vi "Subvi for fastbox.vi"(0 "Cluster in":T1 {"Y axis\nrotation" scale=-32700.0..32700.0; "X axis\nrotation" scale=-32700.0..32700.0; "Z axis" scale=-32700.0..32700.0; "Y axis" scale=-32700.0..32700.0; "X axis" scale=-32700.0..32700.0}, 1 "FPGA VI Reference In":refnum<k20>) -> ()   [LabVIEW 2009]
uses:
  UPD Xbox.ctl
  <vilib>/rvi/interface/nirviReadWriteControl/nirviReadWriteControl.xnode
  FPGA Bitfiles/Athena Brain.lvproj_FPGA Target 2_Combined Steering ~2D.lvbitx
  <vilib>/Utility/error.llb/Error Cluster From Error Code.vi
  <vilib>/rvi/errors/niLvFpgaAdjustHostInterfaceError.vi
  <vilib>/rvi/interface/common/niFpgaNodeNameForErrorReporting.ctl
  <vilib>/rvi/errors/niLvFpgaWhatHappensToTopLevelVI.ctl
  NiRioSrv.dll
panel:
  out "Drive Encoder ft/sec":fxp<+/-,14,4> format="%.12g"
  out "Drive Encoder":i32
  out "Drive Encoder tick/count":i32
  in  "Steering Position Offset":i32
  in  "Steering Proportional Control Feedback Gain":fxp<+/-,20,5> format="%.17g"
  in  "Scale the Steering":dbl
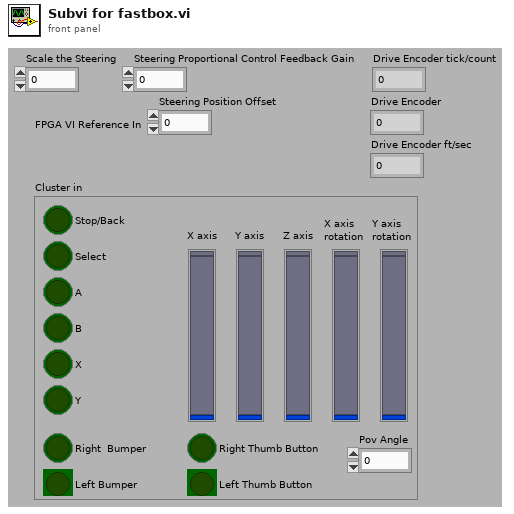
[diagram p1: front panel]
types:
  T1 = typedef "UPD Xbox.ctl" = cluster{"B":bool, "A":bool, "Y":bool, "X":bool, "X axis":i32, "Y axis":i32, "Z axis":i32, "X axis\nrotation":i32, "Y axis\nrotation":i32, "Left Bumper":bool, "Right  Bumper":bool, "Left Thumb Button":bool, "Right Thumb Button":bool, "Stop/Back":bool, "Select":bool, "Pov Angle":i32}
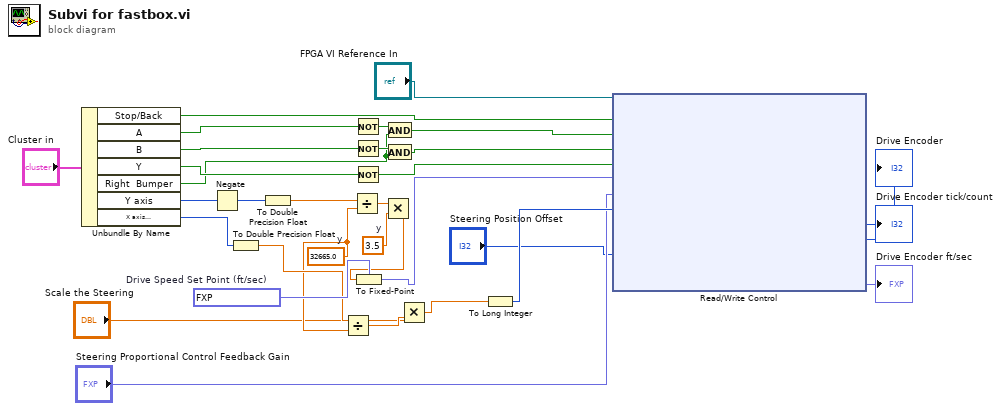
[diagram p0: block diagram]
diagram:
  w11 = 3.5  # y
  w12 = 32665.0  # y
  w29 = fxp<+/-,14,4> 0.0  # Drive Speed Set Point (ft/sec)
  n1 = Unbundle By Name("Cluster in") -> ("Stop/Back"=w31:bool, "A"=w20:bool, "B"=w21:bool, "Y"=w27:bool, "Right  Bumper"=w22:bool, "Y axis"=w30:i32, "X axis\nrotation"=w14:i32)
  n2 = Negate(x=w30) -> (-x=w1:i32)
  n3 = To Double Precision Float(number=w14) -> (double precision float=w13:dbl)
  n4 = To Double Precision Float(number=w1) -> (double precision float=w15:dbl)
  n5 = Divide(x=w13, y=w12) -> (x/y=w10:dbl)
  n6 = Divide(x=w15, y=w12) -> (x/y=w32:dbl)
  n7 = Not(x=w20) -> (.not. x?=w23:bool)
  n8 = Not(x=w21) -> (.not. x?=w24:bool)
  n9 = Not(x=w27) -> (.not. x?=w28:bool)
  n10 = Multiply(x=w32, y=w11) -> (x*y=w17:dbl)
  n11 = To Fixed-Point(fixed-point type=w29, number=w17) -> (fixed-point=w16:fxp<+/-,14,4>)
  n12 = And(x=w23, y=w22) -> (x .and. y?=w25:bool)
  n13 = And(x=w24, y=w22) -> (x .and. y?=w26:bool)
  n14 = Multiply(x="Scale the Steering", y=w10) -> (x*y=w8:dbl)
  n15 = To Long Integer(number=w8) -> (32bit integer=w7:i32)
  n16 = xnode "Read/Write Control"("FPGA VI Reference In"="FPGA VI Reference In", "stop"=w31, "Steering Enable"=w25, "Drive Enable"=w26, "Manual Override?"=w28, "Drive Speed Set Point (ft/sec)"=w16, "Steering Proportional Control Feedback Gain"="Steering Proportional Control Feedback Gain", "Steering Position Target"=w7, "Steering Position Offset"="Steering Position Offset") -> ("Drive Encoder tick/count"=→"Drive Encoder tick/count":i32, "Drive Encoder"=→"Drive Encoder":i32, "Drive Encoder ft/sec"=→"Drive Encoder ft/sec":fxp<+/-,14,4>)  [unwired: 2 in, 2 out]
